vi "Error Query.vi"(8 "error in (no error)":errorcluster, 11 "VISA resource name":refnum<visa-resource-name>) -> (0 "error out":errorcluster, 1 "Error Message":string, 2 "Error Code":i32[](array[numeric]), 3 "VISA resource name out":refnum<visa-resource-name>)   [LabVIEW 2016, in "Agilent 34401.lvlib"]
doc: "This VI queries the instrument for any errors in the instrument's error queue. It will continue to read errors until all errors have been read from the instrument. Any errors will be returned in the Error Out cluster.\n\n<B>Note:</B>\n\nThis VI is called automatically by most driver VIs so it is not usually necessary to call this in an application."
uses:
  <instrlib>/Agilent 34401/Agilent 34401.lvlib
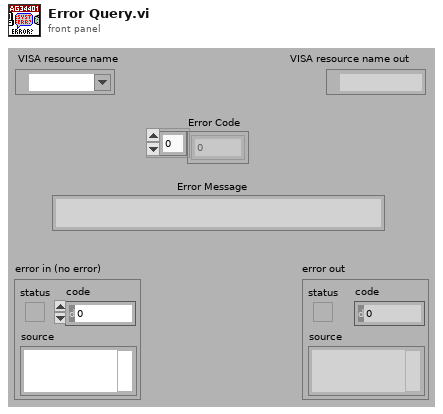
[diagram p1: front panel]
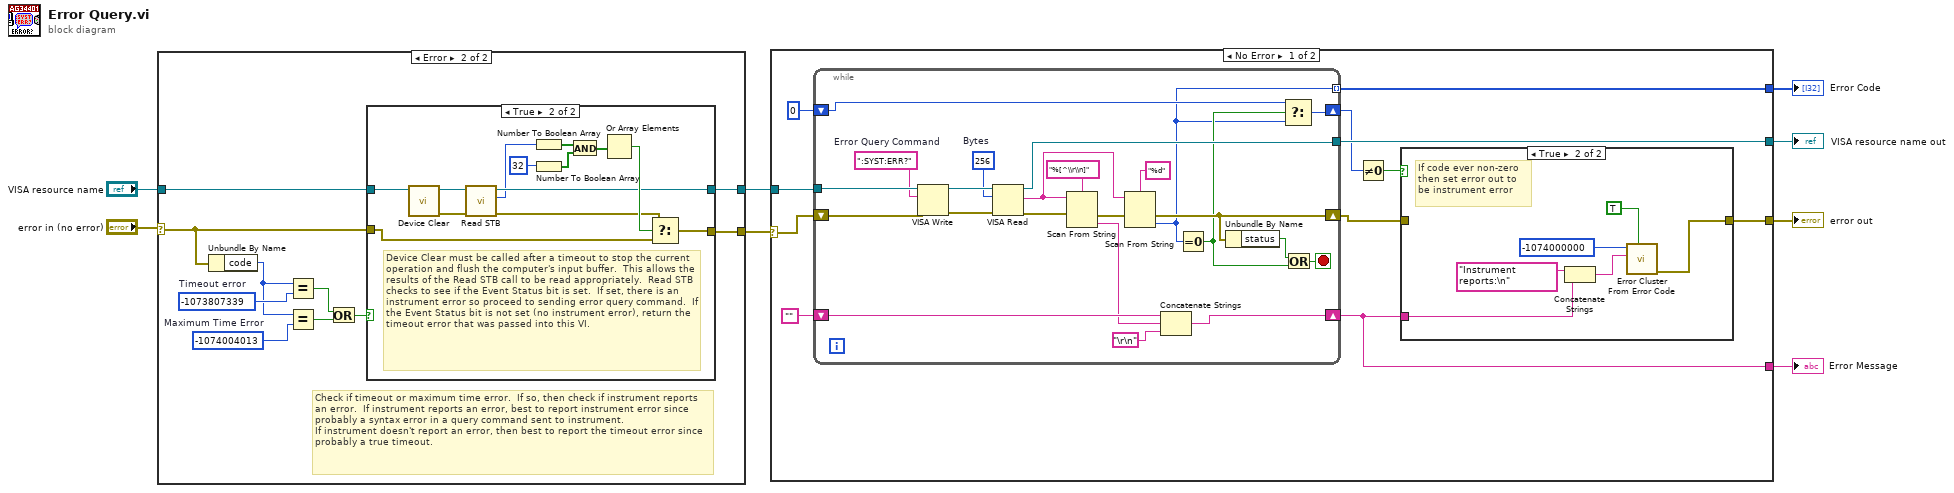
[diagram p0: block diagram]
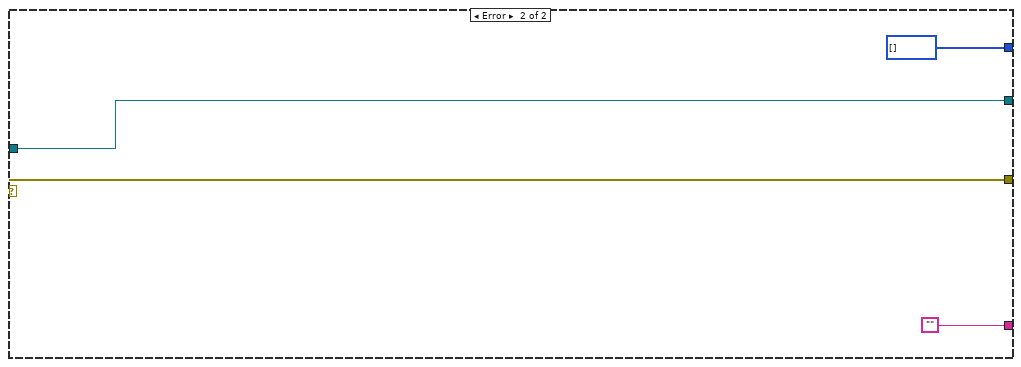
[diagram p5: hidden frame]
diagram:
  n1 = case shown="Error" "error in (no error)" {
    selector: "error in (no error)" -> [w9 w17]
    tunnel: "VISA resource name" -> [w10 w20]
    tunnel: [w10 w18] -> w3
    tunnel: [w9 w16] -> w1
    frame No Error {
    }
    frame Error {
      w14 = -1074004013  # Maximum Time Error
      w19 = -1073807339  # Timeout error
      # "Check if timeout or maximum time error.  If so, then check if instrument reports an error.  If instrument reports an error, best to report instrument error since probably a syntax error in a query command sent to instrument.\nIf instrument doesn't report an error, then best to report the timeout error since probably a true timeout."
      n2 = Unbundle By Name(w17) -> ("code"=w15:i32)
      n3 = Equal?(x=w15, y=w19) -> (x = y?=w11:bool)
      n4 = Equal?(x=w15, y=w14) -> (x = y?=w13:bool)
      n5 = Or(x=w11, y=w13) -> (x .or. y?=w12:bool)
      n6 = case shown="True" w12 {
        tunnel: w20 -> [w22 w28]
        tunnel: [w22 w24] -> w18
        tunnel: w17 -> [w21 w31]
        tunnel: [w21 w30] -> w16
        frame False {
          # "Error code not a timeout, so best to pass on to user."
        }
        frame True {
          # "Device Clear must be called after a timeout to stop the current operation and flush the computer's input buffer.  This allows the results of the Read STB call to be read appropriately.  Read STB checks to see if the Event Status bit is set.  If set, there is an instrument error so proceed to sending error query command.  If the Event Status bit is not set (no instrument error), return the timeout error that was passed into this VI."
          n7 = call <instrlib>:"Device Clear.vi"("VISA Resource Name"=w28) -> ("error out"=w26:errorcluster, "VISA Resource Out"=w27:refnum<visa-resource-name>)  [unwired: 9 in]
          n8 = call <instrlib>:"Read STB.vi"("error in (no error)"=w26, "VISA resource name"=w27) -> ("error out"=w25:errorcluster, "Status Byte"=w23:i32, "VISA resource name out"=w24:refnum<visa-resource-name>)  [unwired: 7 in]
          n9 = Number To Boolean Array(number=w23) -> (Boolean array=w32:bool[])
          n10 = Number To Boolean Array(number=32) -> (Boolean array=w34:bool[])
          n11 = And(x=w32, y=w34) -> (x .and. y?=w33:bool[])
          n12 = Or Array Elements(Boolean array=w33) -> (logical OR=w29:bool)
          n13 = Select(t=w25, s=w29, f=w31) -> (s? t:f=w30:errorcluster)
        }
      }
    }
  }
  n14 = case shown="No Error" w1 {
    selector: w1 -> [w38 w77]
    tunnel: [w46 w80] -> w8
    tunnel: w3 -> [w37 w80]
    tunnel: [w39 w77] -> w6
    tunnel: [w40 "" ("Empty String Constant")] -> w5
    tunnel: [w42 i32[] []] -> w4
    frame No Error {
      n15 = while {
        tunnel: [w76] -> w46
        tunnel: w37 -> [w75]
        shift-right: [w63] -> w40
        shift-left: "" ("Empty String Constant") -> [w66]
        shift-right: [w61] -> w43
        shift-left: 0 -> [w62]
        shift-right: [w59] -> w36
        shift-left: w38 -> [w60]
        tunnel: [w54] -> w42 mode=indexing
        stop <- w69 stop-if-true
        w73 = u32 256  # Bytes
        w71 = ":SYST:ERR?"  # Error Query Command
        n16 = VISA Write(VISA resource name=w75, write buffer=w71, error in (no error)=w60) -> (VISA resource name out=w74:refnum<visa-resource-name>, error out=w72:errorcluster)  [unwired: 1 out]
        n17 = VISA Read(VISA resource name=w74, byte count=w73, error in (no error)=w72) -> (VISA resource name out=w76:refnum<visa-resource-name>, read buffer=w67:string, error out=w58:errorcluster)  [unwired: 1 out]
        n18 = Scan From String(format string="%[^\\r\\n]", input string=w67, error in=w58) -> (error out=w57:errorcluster, output 1=w64:string)  [unwired: 2 in, 2 out]
        n19 = Scan From String(format string="%d", input string=w67, error in=w57) -> (error out=w59:errorcluster, output 1=w54:i32)  [unwired: 2 in, 2 out]
        n20 = Concatenate Strings(w66, w64, "\r\n" ("End of Line Constant")) -> (w63:string)
        n21 = Equal To 0?(x=w54) -> (x = 0?=w55:bool)
        n22 = Unbundle By Name(w59) -> ("status"=w56:bool)
        n23 = Select(t=w62, s=w55, f=w54) -> (s? t:f=w61:i32)
        n24 = Or(x=w56, y=w55) -> (x .or. y?=w69:bool)
      }
      n25 = Not Equal To 0?(x=w43) -> (x != 0?=w41:bool)
      n26 = case shown="True" w41 {
        tunnel: w40 -> [_ w52]
        tunnel: [w47 w48] -> w39
        tunnel: w36 -> [w47 _]
        frame False {
        }
        frame True {
          # "If code ever non-zero\nthen set error out to\nbe instrument error"
          n27 = Concatenate Strings("Instrument reports:\n" ("Source"), w52) -> (w49:string)
          n28 = call <vilib>:"Error Cluster From Error Code.vi"("show call chain? (False)"=TRUE, "error message (\"\")"=w49, "error code (0)"=-1074000000 ("Code")) -> ("error out"=w48:errorcluster)  [unwired: 6 in]
        }
      }
    }
    frame Error {
    }
  }
  "VISA resource name out" <- w8
  "error out" <- w6
  "Error Message" <- w5
  "Error Code" <- w4
